vi "Ex1_4operation.vi"() -> ()   [LabVIEW 2018]
panel:
  out "DIVIDE":dbl
  out "A - B":i8(slide) scale=-9.0..9.0
  out "A * B":i8(knob) scale=0.0..81.0
  in  "B":i8
  out "A / B":dbl(slide) scale=0.0..9.0
  out "A + B":i8
  in  "A":i8(slide) scale=0.0..9.0
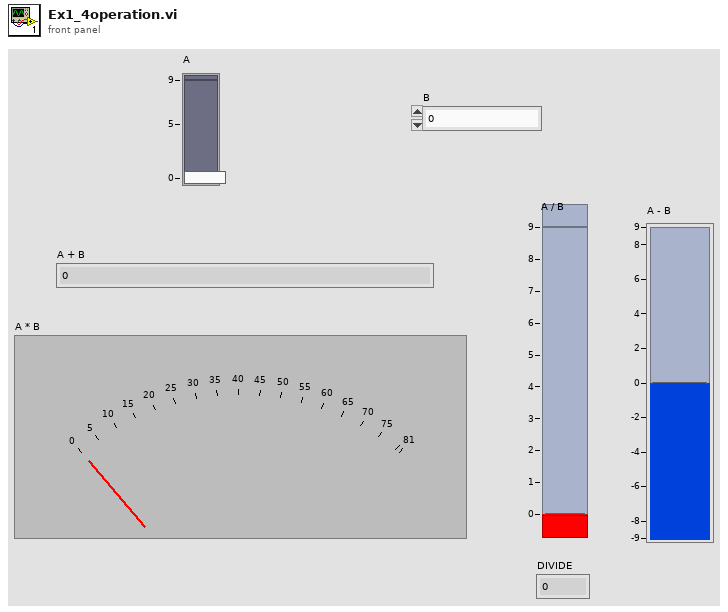
[diagram p1: front panel]
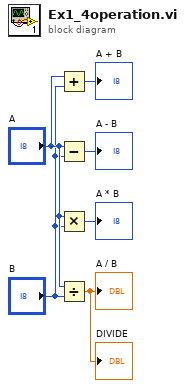
[diagram p0: block diagram]
diagram:
  n1 = Add(x="A", y="B") -> (x+y=→"A + B":i8)
  n2 = Subtract(x="A", y="B") -> (x-y=→"A - B":i8)
  n3 = Multiply(x="A", y="B") -> (x*y=→"A * B":i8)
  n4 = Divide(x="A", y="B") -> (x/y=→"A / B" →"DIVIDE":dbl)
